vi "Test.vi"() -> ()   [LabVIEW 2020, in "Library Instrument & Equipement.lvlib" / "Library FireBase.lvlib" / "Firebase Driver.lvclass"]
uses:
  Firebase Driver.lvclass
  JSON API/JSON Value/Set from JSON string.vi
  JSON API/JSON Value/JSON Value.lvclass
  Firebase Driver.lvclass/Firebase Driver.ctl
  JSON API/Variant JSON/Variant JSON.lvlib
  JSON API/Get Polymorphic/JSON GetSet.lvlib
panel:
  out "Sting_JSON 2":string
  out "error out":errorcluster caption="sortie d'erreur"
  out "données":T1
  out "Link_Last _Document":string
  out "Sting_JSON":string
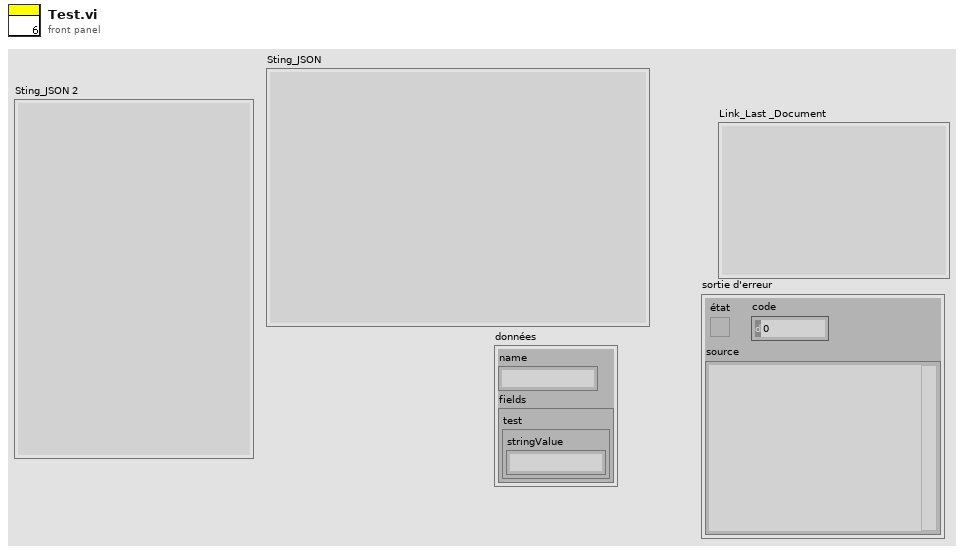
[diagram p1: front panel]
types:
  T1 = cluster{"name":string, "fields":cluster{"test":cluster{"stringValue":string}}}
  T2 = cluster{"fields":cluster{"test":cluster{"stringValue":string}}}
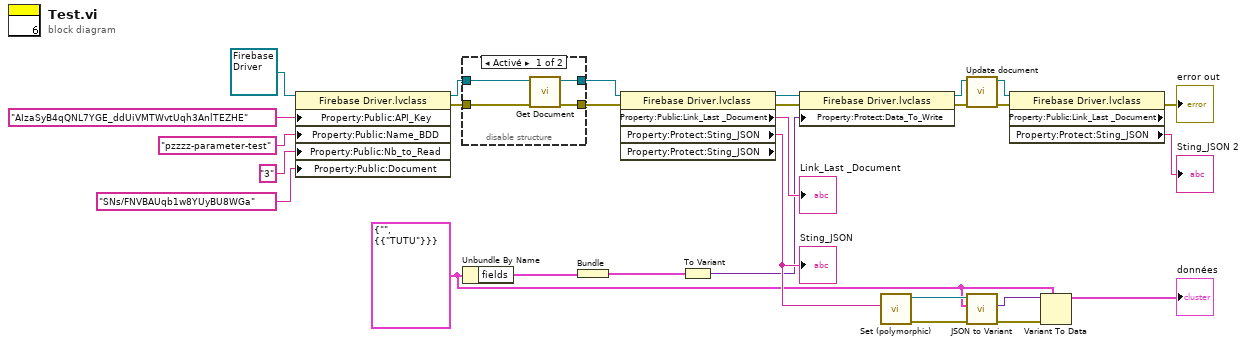
[diagram p0: block diagram]
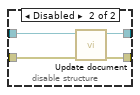
[diagram p2: hidden frame]
diagram:
  w2 = T1 {"name"="", "fields"={"test"={"stringValue"="TUTU"}}} ("document")
  n1 = property class="Firebase Driver.lvclass"(reference=refnum<class "Firebase Driver.lvclass"> refnum ("Firebase (Default) en entrée"), "Property:Public:API_Key"="AIzaSyB4qQNL7YGE_ddUiVMTWvtUqh3AnlTEZHE" ("Input.API_Key"), "Property:Public:Name_BDD"="pzzzz-parameter-test" ("Input.Name_BDD"), "Property:Public:Nb_to_Read"="3" ("Nb_to_Read"), "Property:Public:Document"="SNs/FNVBAUqb1w8YUyBU8WGa" ("Document")) -> (reference out=w25:refnum<class "Firebase Driver.lvclass">, error out=w24:errorcluster)  [unwired: 1 in]
  n2 = disable-structure shown="Activé" {
    disable-tunnel: w25 -> [w32 w33]
    disable-tunnel: w24 -> [w31 w36]
    disable-tunnel: [w30 w34] -> w23
    disable-tunnel: [w29 w35] -> w22
    frame Enabled {
      n3 = call-dynamic "Get Document.vi"("error in (no error)"=w31, "Firebase (Default) en entrée"=w32) -> ("error out"=w29:errorcluster, "Firebase (Default) en sortie"=w30:refnum<class "Firebase Driver.lvclass">)  [unwired: 8 in]
    }
    frame Disabled {
      n4 = call-dynamic "Update document.vi"("error in (no error)"=w36, "Firebase (Default) en entrée"=w33) -> ("error out"=w35:errorcluster, "Firebase (Default) en sortie"=w34:refnum<class "Firebase Driver.lvclass">)  [unwired: 8 in]
    }
  }
  n5 = Unbundle By Name(w2) -> ("fields"=w1:cluster{"test":cluster{"stringValue":string}})
  n6 = Bundle("fields"=w1) -> (w9:T2)  [unwired: 1 in]
  n7 = property class="Firebase Driver.lvclass" props=["Property:Public:Link_Last _Document", "Property:Protect:Sting_JSON", "Property:Protect:Sting_JSON"](reference=w23, error in=w22) -> (reference out=w12:refnum<class "Firebase Driver.lvclass">, error out=w11:errorcluster, "Property:Public:Link_Last _Document"=→"Link_Last _Document":string, "Property:Protect:Sting_JSON"=w14:string)  [unwired: 1 out]
  "Sting_JSON" <- w14
  n8 = To Variant(anything=w9) -> (Variant=w10:variant)
  n9 = property class="Firebase Driver.lvclass"(reference=w12, error in=w11, "Property:Protect:Data_To_Write"=w10) -> (reference out=w7:refnum<class "Firebase Driver.lvclass">, error out=w8:errorcluster)
  n10 = call-poly "Set (polymorphic).vi"("JSON stream"=w14) -> ("error out"=w15:errorcluster, "JSON Value out"=w18:refnum<class "JSON Value.lvclass">)  [unwired: 8 in, 1 out]
  n11 = call-dynamic "Update document.vi"("error in (no error)"=w8, "Firebase (Default) en entrée"=w7) -> ("error out"=w4:errorcluster, "Firebase (Default) en sortie"=w6:refnum<class "Firebase Driver.lvclass">)  [unwired: 8 in]
  n12 = call "JSON to Variant.vi"("error in (no error)"=w15, "Variant (Data Type)"=w2, "JSON Value"=w18) -> ("error out"=w16:errorcluster, "Variant out"=w17:variant)  [unwired: 7 in]
  n13 = property class="Firebase Driver.lvclass" props=["Property:Public:Link_Last _Document", "Property:Protect:Sting_JSON"](reference=w6, error in=w4) -> (error out=→"error out":errorcluster, "Property:Protect:Sting_JSON"=→"Sting_JSON 2":string)  [unwired: 2 out]
  n14 = Variant To Data(error in=w16, type=w2, Variant=w17) -> (data=→"données":T1)  [unwired: 1 out]
